vi "Generate Order Number.vi"(8 "error in (no error)":errorcluster, 11 "Cashier in":refnum<class "Cashier.lvclass">) -> (0 "error out":errorcluster, 2 "Order Number":u32, 3 "Cashier out":refnum<class "Cashier.lvclass">)   [LabVIEW 2020, in "Cashier.lvclass"]
uses:
  Cashier.lvclass
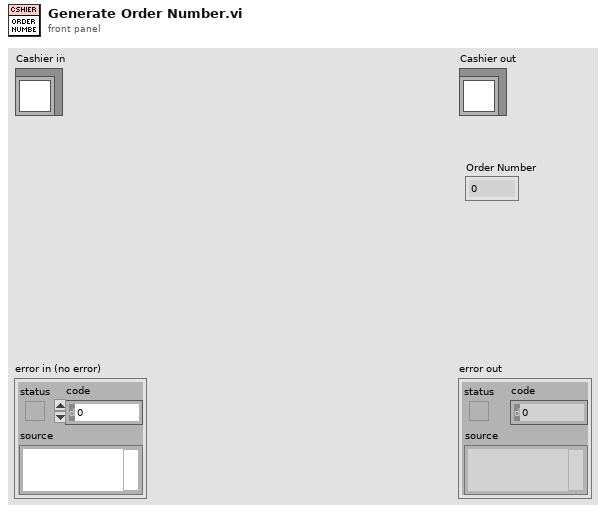
[diagram p1: front panel]
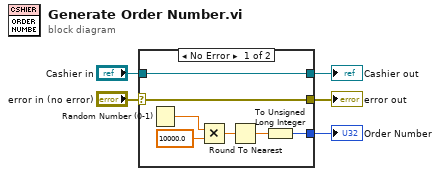
[diagram p0: block diagram]
diagram:
  n1 = case shown="No Error" "error in (no error)" {
    selector: "error in (no error)" -> [w11 w14]
    tunnel: [w11 w14] -> w4
    tunnel: [w12 w13] -> w2
    tunnel: "Cashier in" -> [w12 w13]
    tunnel: [w6 _] -> w1
    frame No Error {
      n2 = Random Number (0-1)() -> (number: 0 to 1=w9:dbl)
      n3 = Multiply(x=w9, y=10000.0) -> (x*y=w10:dbl)
      n4 = Round To Nearest(number=w10) -> (nearest integer value=w7:dbl)
      n5 = To Unsigned Long Integer(number=w7) -> (unsigned 32bit integer=w6:u32)
    }
    frame Error {
    }
  }
  "error out" <- w4
  "Cashier out" <- w2
  "Order Number" <- w1
